vi "数组去零.vi"(1 "输入":dbl[](array[numeric])) -> (0 "输出":dbl[](array[numeric]))   [LabVIEW 2013]
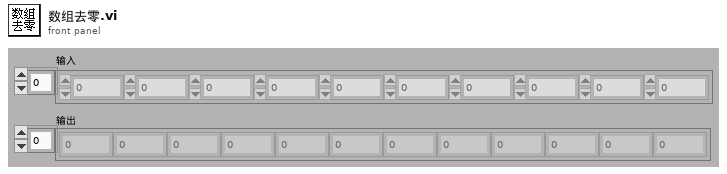
[diagram p1: front panel]
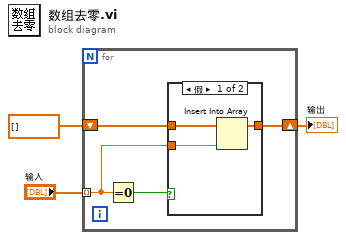
[diagram p0: block diagram]
diagram:
  n1 = for {
    shift-right: [w5] -> w1
    shift-left: dbl[] [] -> [w6]
    tunnel: "输入" -> [w4] mode=indexing
    n2 = Equal To 0?(x=w4) -> (x = 0?=w7:bool)
    n3 = case shown="假" w7 {
      tunnel: w6 -> [w10 w11]
      tunnel: [w9 w11] -> w5
      tunnel: w4 -> [w8 _]
      frame False {
        n4 = Insert Into Array(array=w10, new element=w8) -> (w9:dbl[])  [unwired: 1 in]
      }
      frame True {
      }
    }
  }
  "输出" <- w1
